vi "Build table.vi"(7 "Limit (10k)":i32=10000 format="%.0p", 8 "error in":errorcluster, 9 "Tree Data":refnum<vi>, 10 "New Data in":string[][](array[string]), 11 "Tree Data in":string[][](array[string])) -> (0 "error out":errorcluster, 3 "Tree Data out":string[][](array[string]))   [LabVIEW 2025]
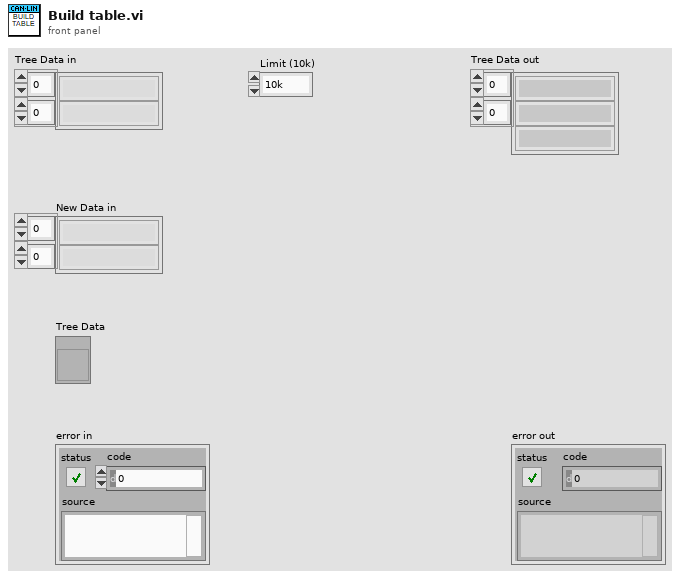
[diagram p1: front panel]
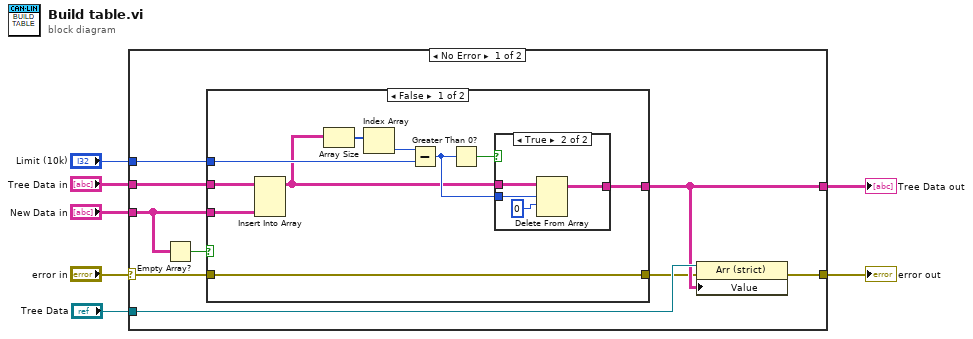
[diagram p0: block diagram]
diagram:
  n1 = case shown="No Error" "error in" {
    selector: "error in" -> [w12 w35]
    tunnel: "New Data in" -> [w15 _]
    tunnel: [w9 w35] -> w5
    tunnel: "Limit (10k)" -> [w14 _]
    tunnel: "Tree Data in" -> [w13 w34]
    tunnel: [w10 w34] -> w2
    tunnel: "Tree Data" -> [w11 _]
    frame No Error {
      n2 = Empty Array?(array=w15) -> (empty?=w16:bool)
      n3 = case shown="False" w16 {
        tunnel: w15 -> [w22 _]
        tunnel: [w19 w33] -> w8
        tunnel: w14 -> [w26 _]
        tunnel: w13 -> [w23 w32]
        tunnel: [w18 w32] -> w10
        tunnel: w12 -> [w19 w33]
        frame False {
          n4 = Insert Into Array(array=w23, new element=w22) -> (w17:string[][])  [unwired: 2 in]
          n5 = Array Size(array=w17) -> (size(s)=w21:i32[])
          n6 = Index Array(array=w21) -> (element=w20:i32)  [unwired: 1 in]
          n7 = Subtract(x=w20, y=w26) -> (x-y=w24:i32)
          n8 = Greater Than 0?(x=w24) -> (x > 0?=w25:bool)
          n9 = case shown="True" w25 {
            tunnel: [w27 w31] -> w18
            tunnel: w24 -> [_ w30]
            tunnel: w17 -> [w27 w28]
            frame False {
            }
            frame True {
              n10 = Delete From Array(array=w28, length=w30, index (row)=0) -> (array with subset deleted=w31:string[][])  [unwired: 1 in, 1 out]
            }
          }
        }
        frame True {
        }
      }
      n11 = property class="Arr (strict)"(reference=w11, error in=w8, "Value"=w10) -> (error out=w9:errorcluster)  [unwired: 1 out]
    }
    frame Error {
    }
  }
  "error out" <- w5
  "Tree Data out" <- w2
